vi "Extract Each Template.vi"(4 "Remaining in":string) -> (6 "Template":string, 7 "Remaining":string)   [LabVIEW 2020, in "HTTP Server.lvlib" / "BasicTemplater.lvclass"]
uses:
  BasicTemplater.lvclass
  BasicTemplater.lvclass/BasicTemplater.ctl
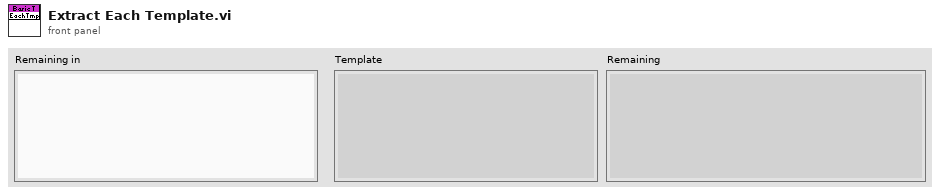
[diagram p1: front panel]
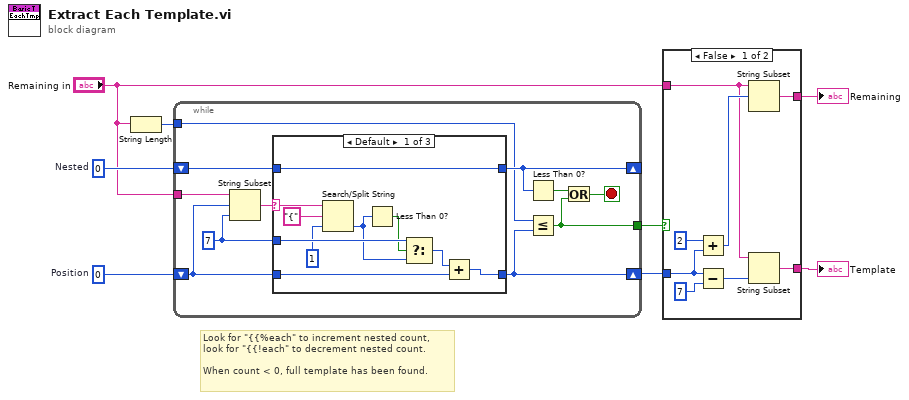
[diagram p0: block diagram]
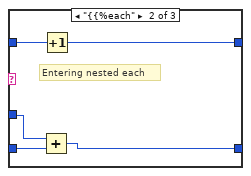
[diagram p3: hidden frame]
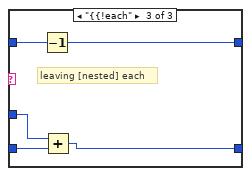
[diagram p4: hidden frame]
diagram:
  w7 = 0  # Position
  w8 = 0  # Nested
  # "Look for \"{{%each\" to increment nested count,\nlook for \"{{!each\" to decrement nested count.\n\nWhen count < 0, full template has been found."
  n1 = String Length(string="Remaining in") -> (length=w6:i32)
  n2 = while {
    shift-right: [w14] -> _
    shift-left: w8 -> [w17]
    shift-right: [w13] -> w4
    shift-left: w7 -> [w15]
    tunnel: "Remaining in" -> [w19]
    tunnel: w6 -> [w12]
    tunnel: [w9] -> w5
    stop <- w10 stop-if-true
    w16 = 7 ("length (rest)")
    n3 = String Subset(string=w19, offset (0)=w15, length (rest)=w16) -> (substring=w18:string)
    n4 = case shown="Default" w18 {
      selector: w18 -> [w28 _ _]
      tunnel: w17 -> [w29 w34 w39]
      tunnel: [w29 w33 w38] -> w14
      tunnel: w16 -> [w26 w31 w36]
      tunnel: w15 -> [w24 w32 w37]
      tunnel: [w22 w30 w35] -> w13
      frame Default {
        n5 = Search/Split String(string=w28, search string/char (-)="{", offset (0)=1) -> (offset of match=w21:i32)  [unwired: 2 out]
        n6 = Less Than 0?(x=w21) -> (x < 0?=w25:bool)
        n7 = Select(t=w26, s=w25, f=w21) -> (s? t:f=w23:i32)
        n8 = Add(x=w23, y=w24) -> (x+y=w22:i32)
      }
      frame "{{%each" {
        # "Entering nested each"
        n9 = Add(x=w31, y=w32) -> (x+y=w30:i32)
        n10 = Increment(x=w34) -> (x+1=w33:i32)
      }
      frame "{{!each" {
        # "leaving [nested] each"
        n11 = Decrement(x=w39) -> (x-1=w38:i32)
        n12 = Add(x=w36, y=w37) -> (x+y=w35:i32)
      }
    }
    n13 = Less Than 0?(x=w14) -> (x < 0?=w11:bool)
    n14 = Less Or Equal?(x=w12, y=w13) -> (x <= y?=w9:bool)
    n15 = Or(x=w11, y=w9) -> (x .or. y?=w10:bool)
  }
  n16 = case shown="False" w5 {
    tunnel: w4 -> [w46 _]
    tunnel: "Remaining in" -> [w41 _]
    tunnel: [w43 _] -> w2
    tunnel: [w40 _] -> w1
    frame False {
      n17 = Add(x=2, y=w46) -> (x+y=w44:i32)
      n18 = Subtract(x=w46, y=7) -> (x-y=w42:i32)
      n19 = String Subset(string=w41, offset (0)=w44) -> (substring=w43:string)  [unwired: 1 in]
      n20 = String Subset(string=w41, length (rest)=w42) -> (substring=w40:string)  [unwired: 1 in]
    }
    frame True {
      # "Mismatched closing {{!each}}"
    }
  }
  "Template" <- w1
  "Remaining" <- w2
